vi "Read Keybind.vi"(9 "Numeric":dbl, 10 "appended array":refnum<vi>[](array[refnum]), 11 "Boolean":bool) -> ()   [LabVIEW 2017]
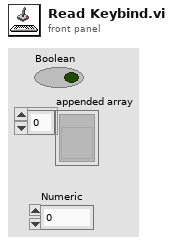
[diagram p1: front panel]
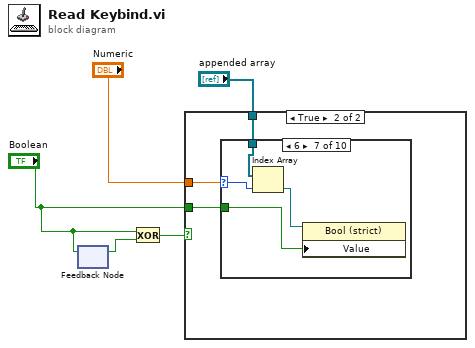
[diagram p0: block diagram]
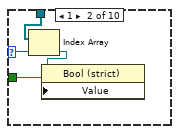
[diagram p4: hidden frame]
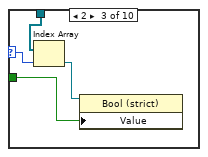
[diagram p5: hidden frame]
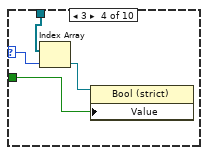
[diagram p6: hidden frame]
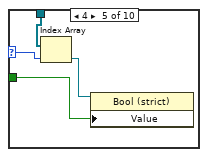
[diagram p7: hidden frame]
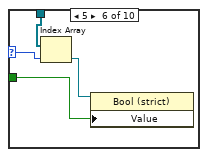
[diagram p8: hidden frame]
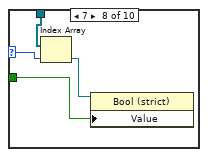
[diagram p9: hidden frame]
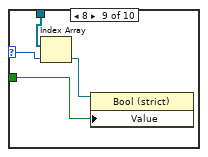
[diagram p10: hidden frame]
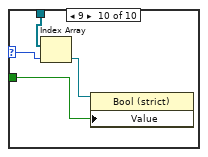
[diagram p11: hidden frame]
diagram:
  n1 = feedback #1() -> (w2:bool)  [unwired: 1 in]
  n2 = feedback-in #1("Boolean") -> ()
  n3 = Exclusive Or(1:w2, 2:"Boolean") -> (0:w3:bool)
  n4 = case shown="True" w3 {
    tunnel: "Boolean" -> [_ w8]
    tunnel: "Numeric" -> [_ w7]
    tunnel: "appended array" -> [_ w6]
    frame False {
    }
    frame True {
      n5 = case shown="6" w7 {
        selector: w7 -> [_ w10 w14 w18 w22 w26 w30 w34 w38 w42]
        tunnel: w8 -> [_ w12 w16 w20 w24 w28 w32 w36 w40 w44]
        tunnel: w6 -> [_ w11 w15 w19 w23 w27 w31 w35 w39 w43]
        frame 0, Default {
        }
        frame 1 {
          n6 = Index Array(array=w11, index=w10) -> (element=w9:refnum<vi>)
          n7 = property class="Bool (strict)"(reference=w9, "Value"=w12) -> ()  [unwired: 1 in, 2 out]
        }
        frame 2 {
          n8 = Index Array(array=w15, index=w14) -> (element=w13:refnum<vi>)
          n9 = property class="Bool (strict)"(reference=w13, "Value"=w16) -> ()  [unwired: 1 in, 2 out]
        }
        frame 3 {
          n10 = Index Array(array=w19, index=w18) -> (element=w17:refnum<vi>)
          n11 = property class="Bool (strict)"(reference=w17, "Value"=w20) -> ()  [unwired: 1 in, 2 out]
        }
        frame 4 {
          n12 = Index Array(array=w23, index=w22) -> (element=w21:refnum<vi>)
          n13 = property class="Bool (strict)"(reference=w21, "Value"=w24) -> ()  [unwired: 1 in, 2 out]
        }
        frame 5 {
          n14 = Index Array(array=w27, index=w26) -> (element=w25:refnum<vi>)
          n15 = property class="Bool (strict)"(reference=w25, "Value"=w28) -> ()  [unwired: 1 in, 2 out]
        }
        frame 6 {
          n16 = Index Array(array=w31, index=w30) -> (element=w29:refnum<vi>)
          n17 = property class="Bool (strict)"(reference=w29, "Value"=w32) -> ()  [unwired: 1 in, 2 out]
        }
        frame 7 {
          n18 = Index Array(array=w35, index=w34) -> (element=w33:refnum<vi>)
          n19 = property class="Bool (strict)"(reference=w33, "Value"=w36) -> ()  [unwired: 1 in, 2 out]
        }
        frame 8 {
          n20 = Index Array(array=w39, index=w38) -> (element=w37:refnum<vi>)
          n21 = property class="Bool (strict)"(reference=w37, "Value"=w40) -> ()  [unwired: 1 in, 2 out]
        }
        frame 9 {
          n22 = Index Array(array=w43, index=w42) -> (element=w41:refnum<vi>)
          n23 = property class="Bool (strict)"(reference=w41, "Value"=w44) -> ()  [unwired: 1 in, 2 out]
        }
      }
    }
  }
